vi "PGC2D Serial Initialize.vi"(8 "error in (no error)":errorcluster, 11 "Array 2":refnum<visa-resource-name>[](array[refnum])) -> (0 "error out":errorcluster, 3 "Array":refnum<visa-resource-name>[](array[refnum]))   [LabVIEW 2019]
uses:
  Program Files (x86)/National Instruments/LabVIEW 2019/examples/Instrument IO/Serial/support/Serial - Settings.ctl
  <vilib>/Instr/_visa.llb/VISA Configure Serial Port (Instr).vi
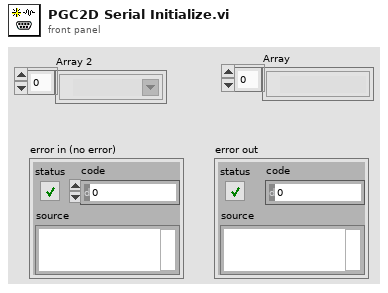
[diagram p1: front panel]
types:
  T1 = typedef "Serial - Settings.ctl" = cluster{"baud rate":u32, "data bits":u16, "parity":enum16{"None", "Odd", "Even", "Mark", "Space"}, "stop bits":u16, "flow control":u16}
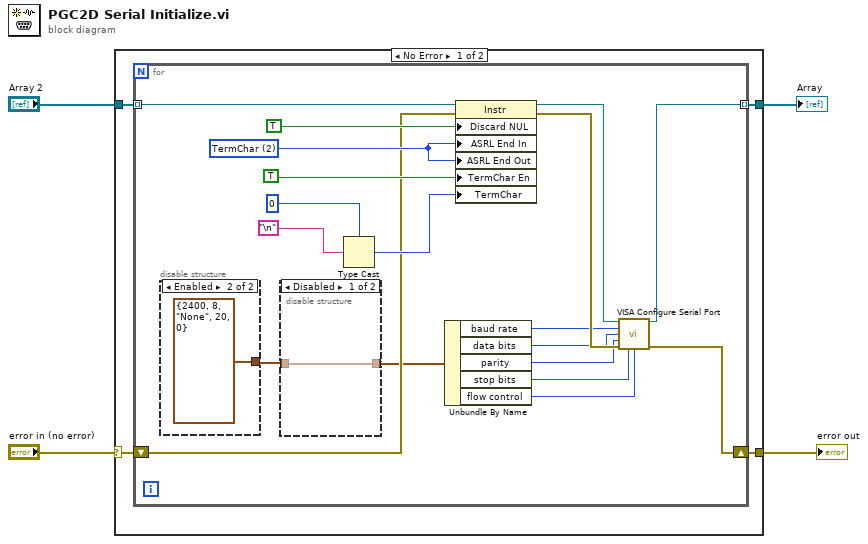
[diagram p0: block diagram]
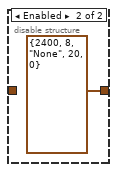
[diagram p3: hidden frame]
diagram:
  n1 = case shown="No Error" "error in (no error)" {
    selector: "error in (no error)" -> [w6 w31]
    tunnel: "Array 2" -> [w5 w32]
    tunnel: [w8 w31] -> w3
    tunnel: [w7 w32] -> w2
    frame No Error {
      n2 = for {
        shift-right: [w14] -> w8
        shift-left: w6 -> [w12]
        tunnel: w5 -> [w11] mode=indexing
        tunnel: [w13] -> w7 mode=indexing
        w20 = u16 2 items=["None", "Last Bit", "TermChar"] ("Serial Settings:End Mode for Reads")
        n3 = disable-structure shown="Enabled" {
          disable-tunnel: [_ T1 {"baud rate"=2400, "data bits"=8, "parity"=enum."None", "stop bits"=20, "flow control"=0} ("input cluster")] -> w9
          frame Disabled {
          }
          frame Enabled {
          }
        }
        n4 = disable-structure shown="Disabled" {
          disable-tunnel: [w29 T1 {"baud rate"=2400, "data bits"=8, "parity"=enum."None", "stop bits"=20, "flow control"=0} ("input cluster")] -> w10
          disable-tunnel: w9 -> [w29 _]
          frame Disabled {
          }
          frame Enabled {
          }
        }
        n5 = Type Cast(type=0, x="\n") -> (*(type *) &x=w23:i32)
        n6 = Unbundle By Name(w10) -> ("baud rate"=w15:u32, "data bits"=w16:u16, "parity"=w17:enum16{"None", "Odd", "Even", "Mark", "Space"}, "stop bits"=w18:u16, "flow control"=w19:u16)
        n7 = property class="Instr"(reference=w11, error in=w12, "Discard NUL"=TRUE ("Serial Settings:Discard NUL Characters"), "ASRL End In"=w20, "ASRL End Out"=w20, "TermChar En"=TRUE ("Message Based Settings:Termination Character Enable"), "TermChar"=w23) -> (reference out=w25:refnum<visa-resource-name>, error out=w24:errorcluster)
        n8 = call-poly "VISA Configure Serial Port"("VISA resource name"=w25, "baud rate (9600)"=w15, "data bits (8)"=w16, "parity (0:none)"=w17, "error in (no error)"=w24, "stop bits (10: 1 bit)"=w18, "flow control (0:none)"=w19) -> ("VISA resource name out"=w13:refnum<visa-resource-name>, "error out"=w14:errorcluster)  [unwired: 7 in]
      }
    }
    frame Error {
    }
  }
  "error out" <- w3
  "Array" <- w2
